vi "JSON TO startup time.vi"(7 "IP":string="192.168.23.100", 8 "error in (no error)":errorcluster, 10 "PORT":dbl=1.0 min=1.0 max=4.0 step=1.0, 11 "MASTER":dbl=1.0 min=1.0 max=10.0 step=1.0) -> (0 "error out":errorcluster, 2 "JSON data":string, 3 "Startup time":u32 format="%^#.10g ms")   [LabVIEW 2022 SP3]
uses:
  <vilib>/JDP Science/JSONtext/JSONtext.lvlib
panel:
  # "Smart conn PWM 100%  duty startup time"
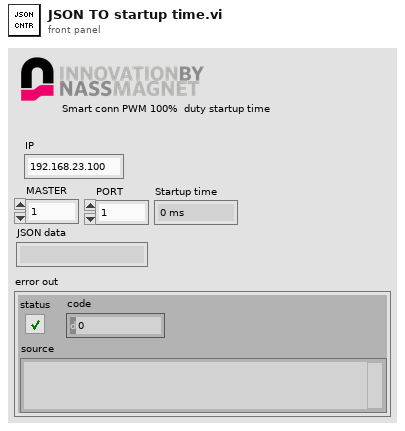
[diagram p1: front panel]
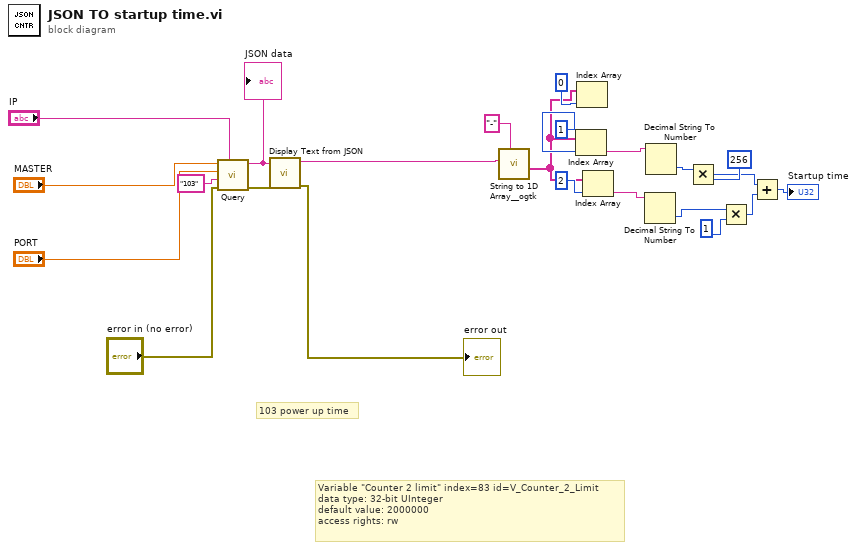
[diagram p0: block diagram]
diagram:
  # "Variable \"Counter 2 limit\" index=83 id=V_Counter_2_Limit\ndata type: 32-bit UInteger\ndefault value: 2000000\naccess rights: rw"
  # "103 power up time"
  n1 = call "Query.vi"("IP"="IP", "error in (no error)"="error in (no error)", "PARAMETERS"="103", "PORT"="PORT", "MASTER"="MASTER") -> ("error out"=w13:errorcluster, "Response"=w23:string)  [unwired: 5 in]
  "JSON data" <- w23
  n2 = call <vilib>:"Display Text from JSON.vi"("error in (no error)"=w13, "Input JSON"=w23) -> ("error out"=→"error out":errorcluster, "Display Text"=w6:string)  [unwired: 7 in, 1 out]
  n3 = call <userlib>:"String to 1D Array__ogtk.vi"("delimiter (Tab)"="-", "string"=w6) -> ("Array of Strings"=w17:string[])  [unwired: 9 in]
  n4 = Index Array(array=w17, index=1) -> (element=w7:string)
  n5 = Index Array(array=w17, index=0) -> ()  [unwired: 1 out]
  n6 = Index Array(array=w17, index=2) -> (element=w8:string)
  n7 = Decimal String To Number(string=w8) -> (number=w10:i32)  [unwired: 2 in, 1 out]
  n8 = Decimal String To Number(string=w7) -> (number=w4:i32)  [unwired: 2 in, 1 out]
  n9 = Multiply(x=w4, y=u32 256) -> (x*y=w5:u32)
  n10 = Multiply(x=w10, y=u32 1) -> (x*y=w9:u32)
  n11 = Add(x=w5, y=w9) -> (x+y=→"Startup time":u32)
